vi "Device info to text.vi"(0 "chanInfo out":T1={"Flags"=2, "Type"=8, "ID"=67330068, "LocId"=87, "SerialNumber[0]"=70, "SerialNumber[1]"=84, "SerialNumber[2]"=88, "SerialNumber[3]"=81, "SerialNumber[4]"=67, "SerialNumber[5]"=77, "SerialNumber[6]"=80, "SerialNumber[7]"=90, "SerialNumber[8]"=0, "SerialNumber[9]"=0, "SerialNumber[10]"=0, "SerialNumber[11]"=0, "SerialNumber[12]"=56, "SerialNumber[13]"=-13, "SerialNumber[14]"=18, "SerialNumber[15]"=0, "Description[0]"=67, "Description[1]"=50, "Description[2]"=51, "Description[3]"=50, "Description[4]"=72, "Description[5]"=77, "Description[6]"=45, "Description[7]"=68, "Description[8]"=68, "Description[9]"=72, "Description[10]"=83, "Description[11]"=76, "Description[12]"=45, "Description[13]"=48, "Description[14]"=0, "Description[15]"=0, "Description[16]"=12, "Description[17]"=-13, "Description[18]"=18, "Description[19]"=0, "Description[20]"=122, "Description[21]"=-104, "Description[22]"=-69, "Description[23]"=117, "Description[24]"=96, "Description[25]"=79, "Description[26]"=0, "Description[27]"=0, "Description[28]"=72, "Description[29]"=-13, "Description[30]"=18, "Description[31]"=0, "Description[32]"=108, "Description[33]"=-89, "Description[34]"=-69, "Description[35]"=117, "Description[36]"=-110, "Description[37]"=-89, "Description[38]"=-69, "Description[39]"=117, "Description[40]"=4, "Description[41]"=-122, "Description[42]"=75, "Description[43]"=121, "Description[44]"=-52, "Description[45]"=-90, "Description[46]"=-69, "Description[47]"=117, "Description[48]"=-88, "Description[49]"=31, "Description[50]"=46, "Description[51]"=16, "Description[52]"=1, "Description[53]"=0, "Description[54]"=0, "Description[55]"=0, "Description[56]"=2, "Description[57]"=0, "Description[58]"=0, "Description[59]"=0, "Description[60]"=0, "Description[61]"=0, "Description[62]"=0, "Description[63]"=0, "ftHandle"=0}) -> (4 "Serial number":string, 6 "Description":string)   [LabVIEW 2024, in "libMPSSE-I2C.lvlib"]
doc: "This Vi convert the data cluster to text."
uses:
  libMPSSE-I2C.lvlib
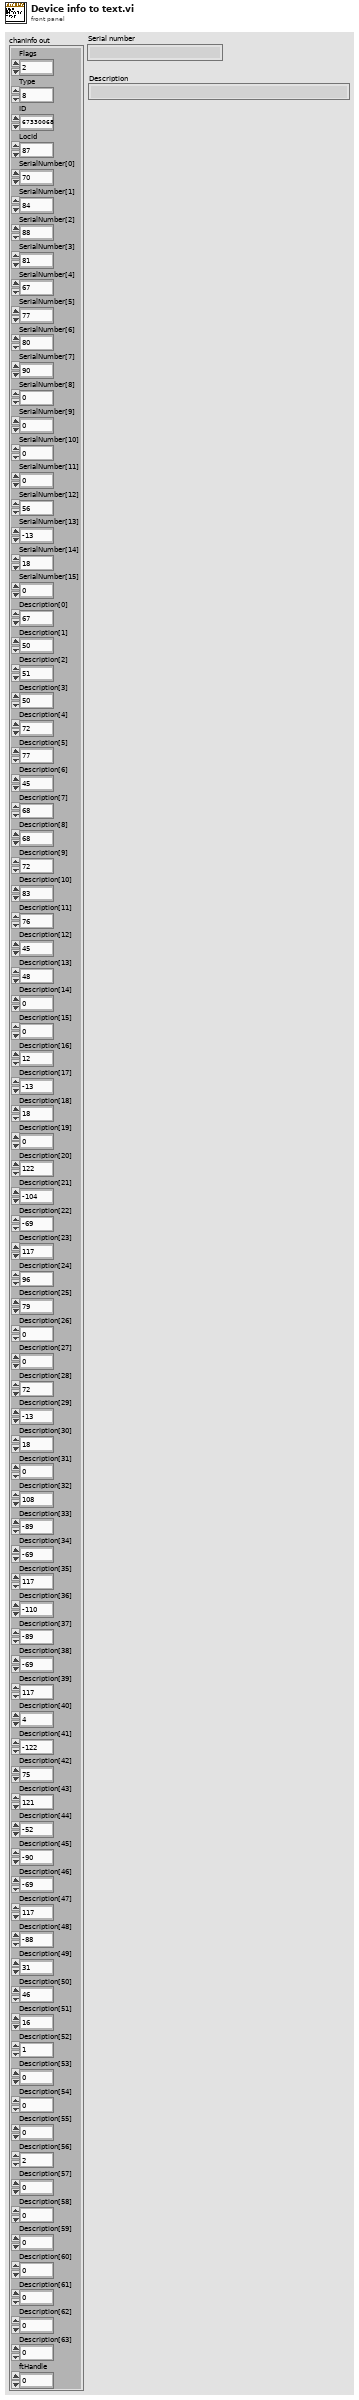
[diagram p1: front panel]
types:
  T1 = cluster{"Flags":u32, "Type":u32, "ID":u32, "LocId":u32, "SerialNumber[0]":i8, "SerialNumber[1]":i8, "SerialNumber[2]":i8, "SerialNumber[3]":i8, "SerialNumber[4]":i8, "SerialNumber[5]":i8, "SerialNumber[6]":i8, "SerialNumber[7]":i8, "SerialNumber[8]":i8, "SerialNumber[9]":i8, "SerialNumber[10]":i8, "SerialNumber[11]":i8, "SerialNumber[12]":i8, "SerialNumber[13]":i8, "SerialNumber[14]":i8, "SerialNumber[15]":i8, "Description[0]":i8, "Description[1]":i8, "Description[2]":i8, "Description[3]":i8, "Description[4]":i8, "Description[5]":i8, "Description[6]":i8, "Description[7]":i8, "Description[8]":i8, "Description[9]":i8, "Description[10]":i8, "Description[11]":i8, "Description[12]":i8, "Description[13]":i8, "Description[14]":i8, "Description[15]":i8, "Description[16]":i8, "Description[17]":i8, "Description[18]":i8, "Description[19]":i8, "Description[20]":i8, "Description[21]":i8, "Description[22]":i8, "Description[23]":i8, "Description[24]":i8, "Description[25]":i8, "Description[26]":i8, "Description[27]":i8, "Description[28]":i8, "Description[29]":i8, "Description[30]":i8, "Description[31]":i8, "Description[32]":i8, "Description[33]":i8, "Description[34]":i8, "Description[35]":i8, "Description[36]":i8, "Description[37]":i8, "Description[38]":i8, "Description[39]":i8, "Description[40]":i8, "Description[41]":i8, "Description[42]":i8, "Description[43]":i8, "Description[44]":i8, "Description[45]":i8, "Description[46]":i8, "Description[47]":i8, "Description[48]":i8, "Description[49]":i8, "Description[50]":i8, "Description[51]":i8, "Description[52]":i8, "Description[53]":i8, "Description[54]":i8, "Description[55]":i8, "Description[56]":i8, "Description[57]":i8, "Description[58]":i8, "Description[59]":i8, "Description[60]":i8, "Description[61]":i8, "Description[62]":i8, "Description[63]":i8, "ftHandle":u32}
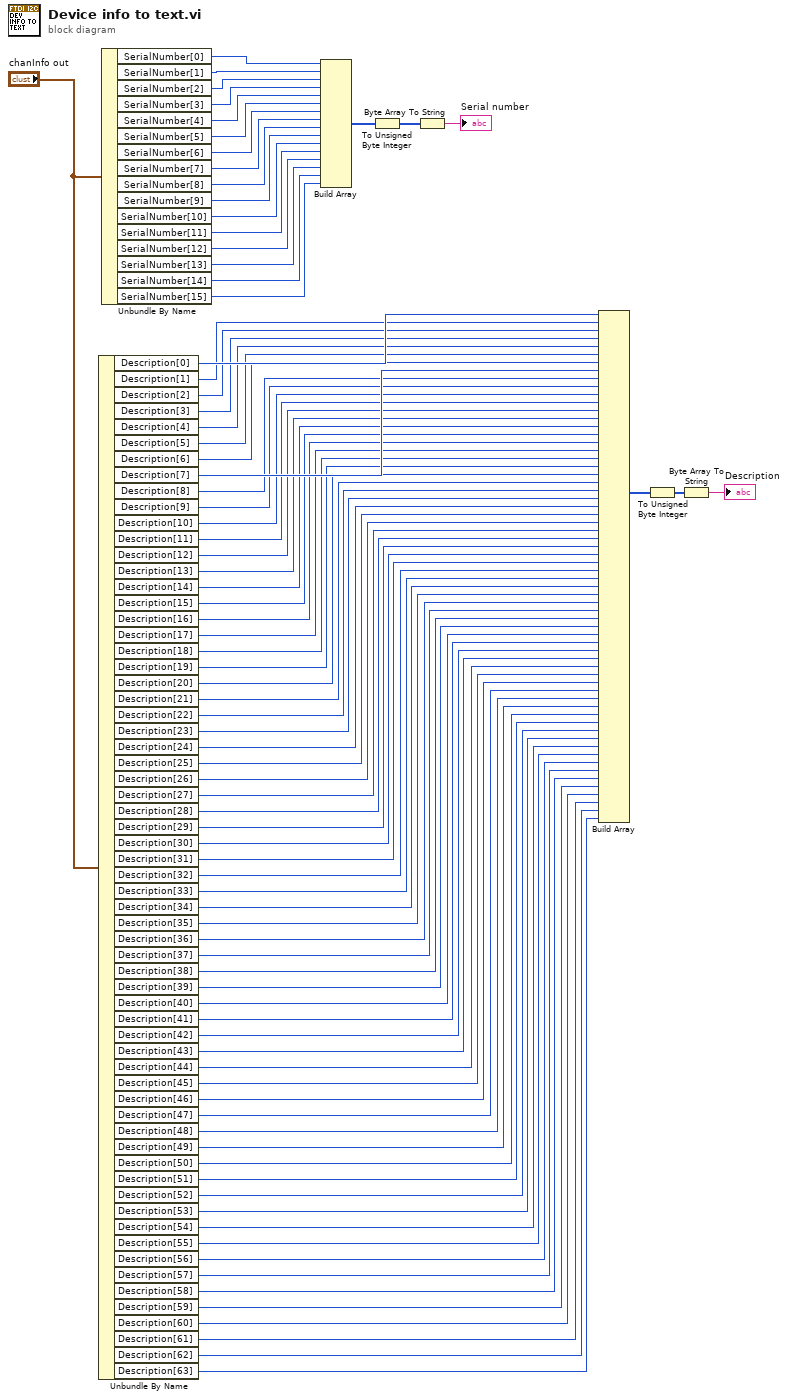
[diagram p0: block diagram]
diagram:
  n1 = Unbundle By Name("chanInfo out") -> ("Description[0]"=w69:i8, "Description[1]"=w68:i8, "Description[2]"=w67:i8, "Description[3]"=w66:i8, "Description[4]"=w65:i8, "Description[5]"=w64:i8, "Description[6]"=w63:i8, "Description[7]"=w62:i8, "Description[8]"=w61:i8, "Description[9]"=w60:i8, "Description[10]"=w59:i8, "Description[11]"=w58:i8, "Description[12]"=w57:i8, "Description[13]"=w56:i8, "Description[14]"=w55:i8, "Description[15]"=w54:i8, "Description[16]"=w50:i8, "Description[17]"=w49:i8, "Description[18]"=w48:i8, "Description[19]"=w47:i8, "Description[20]"=w46:i8, "Description[21]"=w45:i8, "Description[22]"=w44:i8, "Description[23]"=w43:i8, "Description[24]"=w42:i8, "Description[25]"=w41:i8, "Description[26]"=w40:i8, "Description[27]"=w39:i8, "Description[28]"=w38:i8, "Description[29]"=w37:i8, "Description[30]"=w36:i8, "Description[31]"=w35:i8, "Description[32]"=w34:i8, "Description[33]"=w33:i8, "Description[34]"=w32:i8, "Description[35]"=w31:i8, "Description[36]"=w30:i8, "Description[37]"=w29:i8, "Description[38]"=w28:i8, "Description[39]"=w27:i8, "Description[40]"=w26:i8, "Description[41]"=w25:i8, "Description[42]"=w24:i8, "Description[43]"=w23:i8, "Description[44]"=w22:i8, "Description[45]"=w21:i8, "Description[46]"=w20:i8, "Description[47]"=w19:i8, "Description[48]"=w18:i8, "Description[49]"=w17:i8, "Description[50]"=w16:i8, "Description[51]"=w15:i8, "Description[52]"=w14:i8, "Description[53]"=w13:i8, "Description[54]"=w12:i8, "Description[55]"=w11:i8, "Description[56]"=w10:i8, "Description[57]"=w9:i8, "Description[58]"=w8:i8, "Description[59]"=w7:i8, "Description[60]"=w6:i8, "Description[61]"=w5:i8, "Description[62]"=w4:i8, "Description[63]"=w3:i8)
  n2 = Unbundle By Name("chanInfo out") -> ("SerialNumber[0]"=w87:i8, "SerialNumber[1]"=w86:i8, "SerialNumber[2]"=w85:i8, "SerialNumber[3]"=w84:i8, "SerialNumber[4]"=w83:i8, "SerialNumber[5]"=w82:i8, "SerialNumber[6]"=w81:i8, "SerialNumber[7]"=w80:i8, "SerialNumber[8]"=w79:i8, "SerialNumber[9]"=w78:i8, "SerialNumber[10]"=w77:i8, "SerialNumber[11]"=w76:i8, "SerialNumber[12]"=w75:i8, "SerialNumber[13]"=w74:i8, "SerialNumber[14]"=w73:i8, "SerialNumber[15]"=w72:i8)
  n3 = Build Array(w87, w86, w85, w84, w83, w82, w81, w80, w79, w78, w77, w76, w75, w74, w73, w72) -> (w71:i8[])
  n4 = To Unsigned Byte Integer(number=w71) -> (unsigned 8bit integer=w2:u8[])
  n5 = Byte Array To String(unsigned byte array=w2) -> (string=→"Serial number":string)
  n6 = Build Array(w69, w68, w67, w66, w65, w64, w63, w62, w61, w60, w59, w58, w57, w56, w55, w54, w50, w49, w48, w47, w46, w45, w44, w43, w42, w41, w40, w39, w38, w37, w36, w35, w34, w33, w32, w31, w30, w29, w28, w27, w26, w25, w24, w23, w22, w21, w20, w19, w18, w17, w16, w15, w14, w13, w12, w11, w10, w9, w8, w7, w6, w5, w4, w3) -> (w53:i8[])
  n7 = To Unsigned Byte Integer(number=w53) -> (unsigned 8bit integer=w1:u8[])
  n8 = Byte Array To String(unsigned byte array=w1) -> (string=→"Description":string)
